vi "File_FromClass.vi"(8 "error in (no error)":errorcluster, 10 "File.lvclass":refnum<class "File.lvclass">, 11 "Node Ptr":T1 format="%.0x") -> (0 "error out":errorcluster, 3 "Node Ptr Out":T1 format="%.0x")   [LabVIEW 2024, in "Embedded TDMS Logger System Explorer.lvlib"]
doc: "Updates the file properties in the VeriStand System Definition File Custom Device based on a given File definition and subsequently populates the group sections and channels defined as children of this class."
uses:
  Embedded TDMS Logger System Explorer.lvlib
  Shared/File Classes/File/File.lvclass
  <vilib>/NI VeriStand/Custom Device API/Custom Device Item Ref.ctl
  <vilib>/NI VeriStand/Custom Device API/Set Item Property (String).vi
  <vilib>/NI VeriStand/Custom Device API/Set Item Property (Variant).vi
  <vilib>/NI VeriStand/Custom Device API/Custom Device API.lvlib
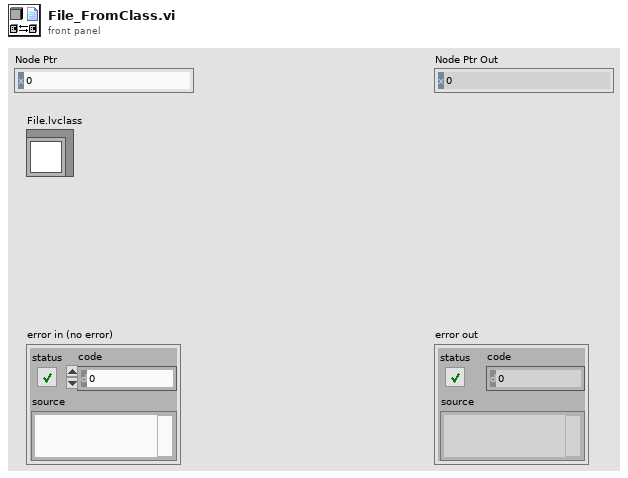
[diagram p1: front panel]
types:
  T1 = typedef "Custom Device API.lvlib/Custom Device Item Ref.ctl" = u64
  T2 = typedef "Meta Data.ctl" = cluster{"Key":string, "Value":string}
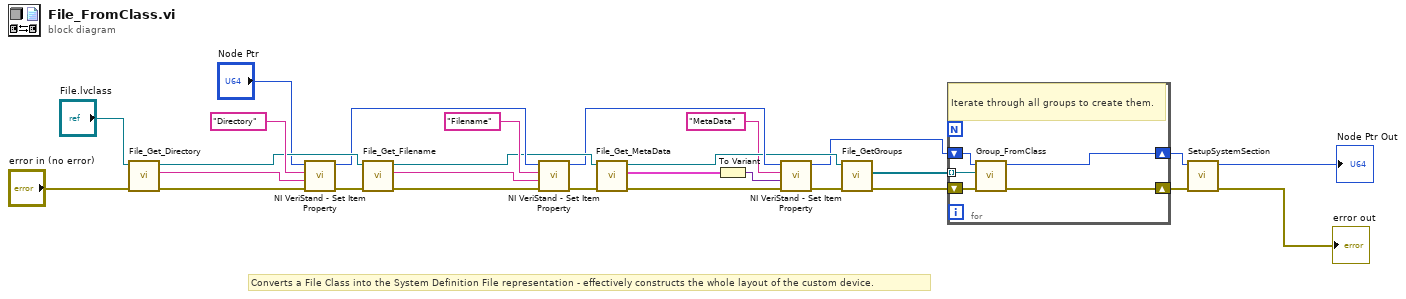
[diagram p0: block diagram]
diagram:
  # "Converts a File Class into the System Definition File representation - effectively constructs the whole layout of the custom device."
  n1 = call-dynamic "File_Get_Directory.vi"("error in (no error)"="error in (no error)", "File in"="File.lvclass") -> ("error out"=w25:errorcluster, "Directory"=w26:string, "File out"=w22:refnum<class "File.lvclass">)  [unwired: 7 in]
  n2 = call-poly <vilib>:"NI VeriStand - Set Item Property.vi"("error in (no error)"=w25, "Value"=w26, "Property Name"="Directory", "Item Ref in"="Node Ptr") -> ("error out"=w21:errorcluster, "Item Ref out"=w20:T1)  [unwired: 5 in, 1 out]
  n3 = call-dynamic "File_Get_Filename.vi"("error in (no error)"=w21, "File in"=w22) -> ("error out"=w18:errorcluster, "Name"=w19:string, "File out"=w15:refnum<class "File.lvclass">)  [unwired: 7 in]
  n4 = call-poly <vilib>:"NI VeriStand - Set Item Property.vi"("error in (no error)"=w18, "Value"=w19, "Property Name"="Filename", "Item Ref in"=w20) -> ("error out"=w14:errorcluster, "Item Ref out"=w13:T1)  [unwired: 5 in, 1 out]
  n5 = call-dynamic "File_Get_MetaData.vi"("error in (no error)"=w14, "File in"=w15) -> ("error out"=w12:errorcluster, "Meta Data"=w17:T2[], "File out"=w11:refnum<class "File.lvclass">)  [unwired: 7 in]
  n6 = To Variant(anything=w17) -> (Variant=w16:variant)
  n7 = call-poly <vilib>:"NI VeriStand - Set Item Property.vi"("error in (no error)"=w12, "Value"=w16, "Property Name"="MetaData", "Item Ref in"=w13) -> ("error out"=w10:errorcluster, "Item Ref out"=w7:T1)  [unwired: 5 in, 1 out]
  n8 = call-dynamic "File_GetGroups.vi"("error in (no error)"=w10, "File in"=w11) -> ("error out"=w8:errorcluster, "Groups"=w9:refnum<class "Group.lvclass">[])  [unwired: 7 in, 1 out]
  n9 = for {
    tunnel: w9 -> [w30] mode=indexing
    shift-right: [w31] -> w1
    shift-left: w8 -> [w32]
    shift-right: [w29] -> w4
    shift-left: w7 -> [w33]
    # "Iterate through all groups to create them."
    n10 = call "Group_FromClass.vi"("error in (no error)"=w32, "Group.lvclass"=w30, "Node Ptr"=w33) -> ("error out"=w31:errorcluster, "Node Ptr Out"=w29:T1)  [unwired: 6 in, 1 out]
  }
  n11 = call "SetupSystemSection.vi"("error in (no error)"=w1, "Node Ptr"=w4) -> ("error out"=→"error out":errorcluster, "Parent Ref Out"=→"Node Ptr Out":T1)  [unwired: 4 in, 4 out]
